vi "Read MediatorBusMonitor Type.vi"(11 "IMediator in":refnum<class "IMediator.lvclass">) -> (2 "MediatorBusMonitor (Type)":refnum<class "IMediatorBusMonitor.lvclass">)   [LabVIEW 2017, in "IMediator.lvlib" / "IMediator.lvclass"]
uses:
  IMediator.lvclass
  IMediatorBusMonitor/MediatorBusMonitor/IMediatorBusMonitor.lvclass
  IMediator.lvclass/IMediator.ctl
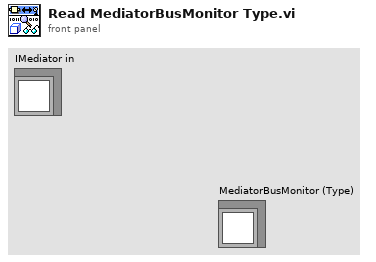
[diagram p1: front panel]
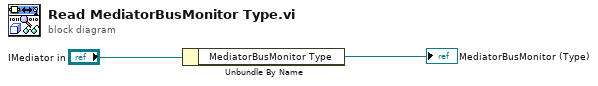
[diagram p0: block diagram]
diagram:
  n1 = Unbundle By Name("IMediator in") -> ("MediatorBusMonitor Type"=→"MediatorBusMonitor (Type)":refnum<class "IMediatorBusMonitor.lvclass">)
